vi "ColorProcessing2016_Custom2.vi"(11 "Original":T5=refnum) -> (0 "Blob array":T2(array[cluster])=[{"Area"=410.0, "Object Info"={"Object Center"={"X"=155.50975, "Y"=158.86829}, "Bounding Box"={"X Left"=142, "Y Top"=150, "X Right"=169, "Y Bottom"=168}, "Area"=410.0, "Orientation"=9.943739, "Aspect Ratio"=1.5, "Nb Holes"=0}}], 1 "Masked":T5(plugin-control), 2 "Targets":T4[](array[typedef]), 3 "Original Image":T5(plugin-control), 4 "Scored Particle Info 2":T1(array[cluster]))   [LabVIEW 2015]
uses:
  Camera Types.ctl
  <vilib>/vision/Image Controls.llb/IMAQ Image.ctl
  Scores.ctl
  <vilib>/vision/NI_Vision_Development_Module.lvlib
panel:
  in  "Range":cluster{"Lower value":sgl, "Upper value":sgl}={"Lower value"=128.0, "Upper value"=255.0} {"Upper value" format="%.2f"; "Lower value" format="%.2f"}
  in  "Particle Count Limit":i32=3
  out "Scored Particle Info":T1(array[cluster])
  in  "Area Size Limit %":dbl=0.5
  in  "Settings":T3={"Objects"=0, "Threshold"=1, "Reject Border"=TRUE, "Fill Holes"=FALSE, "Min Object Size"=TRUE, "Min Size"=350, "Max Object Size"=TRUE, "Max Size"=700, "Show Search Area"=TRUE, "Show Center"=TRUE, "Show Bounding Box"=TRUE} {"Objects" items=["Bright Objects", "Dark Objects"]; "Threshold" min=1 max=999999999 step=1; "Max Size" min=1 max=999999999 step=1; "Min Size" min=1 max=999999999 step=1}
  out "Qualified Particles":i32=3
  out "Sorted Particle Scores":T6(array[cluster]) {"Center" format="%#_3g"; "Moment Factor" format="%#_3g"; "Aspect Ratio" format="%#_3g"; "Area to CH" format="%#_3g"; "X" format="%#_3g"; "Y" format="%#_3g"}
  out "Detected Targets":T7(array[cluster]) {"Normalized Rect"."Numeric 5" format="%#_2g"; "Normalized Rect"."Numeric 3" format="%#_2g"; "Normalized Rect"."Numeric 2" format="%#_2g"; "Normalized Rect"."Numeric" format="%#_2g"}
  in  "Aspect Ratio Fudge Factor":dbl=1.0
  out "Highest Avg Score":dbl=85.32840563115018 format="%#_3g"
  in  "Min Score Threshold":i32=70
  in  "Camera Type":T8=enum."MS HD3000 square"
  in  "ROI DescriptorEmphasize Limit Tests":bool=TRUE
  # "Density Profile"
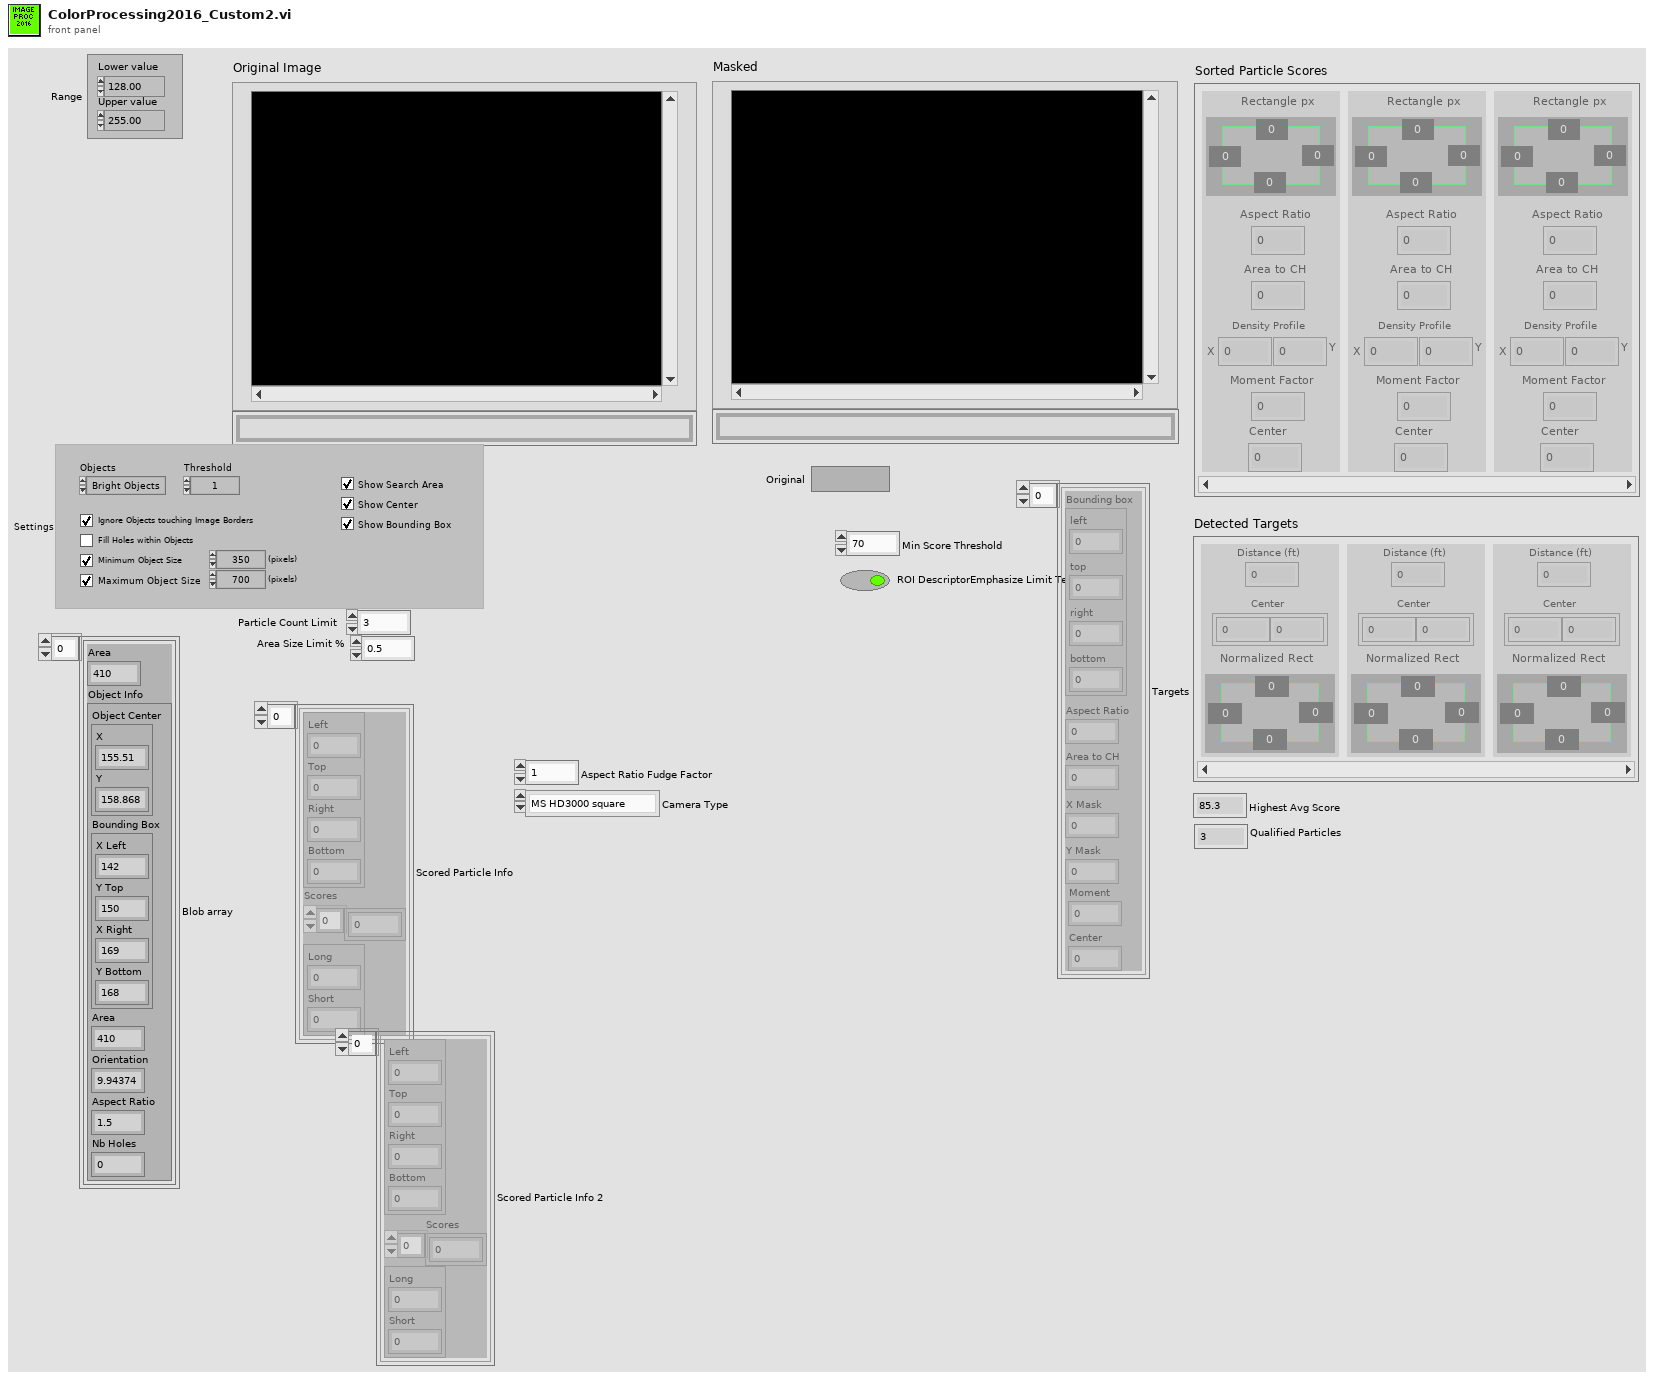
[diagram p1: front panel]
types:
  T1 = cluster{cluster{"Left":dbl, "Top":dbl, "Right":dbl, "Bottom":dbl}, "Scores":dbl[], cluster{"Long":dbl, "Short":dbl}}[]
  T2 = cluster{"Area":sgl, "Object Info":cluster{"Object Center":cluster{"X":sgl, "Y":sgl}, "Bounding Box":cluster{"X Left":i32, "Y Top":i32, "X Right":i32, "Y Bottom":i32}, "Area":sgl, "Orientation":sgl, "Aspect Ratio":sgl, "Nb Holes":i32}}[]
  T3 = cluster{"Objects":u16, "Threshold":i32, "Reject Border":bool, "Fill Holes":bool, "Min Object Size":bool, "Min Size":i32, "Max Object Size":bool, "Max Size":i32, "Show Search Area":bool, "Show Center":bool, "Show Bounding Box":bool}
  T4 = typedef "Scores.ctl" = cluster{"Bounding box":cluster{"left":dbl, "top":dbl, "right":dbl, "bottom":dbl}, "Aspect Ratio":dbl, "Area to CH":dbl, "X Mask":dbl, "Y Mask":dbl, "Moment":dbl, "Center":dbl}
  T5 = typedef "IMAQ Image.ctl" = refnum<image>
  T6 = cluster{"Rectangle px":cluster{"Numeric":dbl, "Numeric 2":dbl, "Numeric 3":dbl, "Numeric 5":dbl}, "Aspect Ratio":dbl, "Area to CH":dbl, "X":dbl, "Y":dbl, "Moment Factor":dbl, "Center":dbl}[]
  T7 = cluster{"Distance (ft)":dbl, "Center":cluster{dbl, dbl}, "Normalized Rect":cluster{"Numeric":dbl, "Numeric 2":dbl, "Numeric 3":dbl, "Numeric 5":dbl}}[]
  T8 = typedef "Camera Types.ctl" = enum16{"206", "1011", "1013", "MS HD3000 square", "MS HD3000 640x480"}
  T9 = typedef "Particle Parameters" = i32
  T10 = typedef "IMAQ Rectangle" = cluster{"Left":i32, "Top":i32, "Right":i32, "Bottom":i32, "Rotation":dbl}
  T11 = typedef "Image Type" = u32
  T12 = cluster{"Object Center":cluster{"X":sgl, "Y":sgl}, "Bounding Box":cluster{"X Left":i32, "Y Top":i32, "X Right":i32, "Y Bottom":i32}, "Area":sgl, "Orientation":sgl, "Aspect Ratio":sgl, "Nb Holes":i32}[]
  T13 = cluster{"Area":sgl, "Object Info":cluster{"Object Center":cluster{"X":sgl, "Y":sgl}, "Bounding Box":cluster{"X Left":i32, "Y Top":i32, "X Right":i32, "Y Bottom":i32}, "Area":sgl, "Orientation":sgl, "Aspect Ratio":sgl, "Nb Holes":i32}}
  T14 = cluster{"Rectangle":cluster{"Numeric":dbl, "Numeric 2":dbl, "Numeric 3":dbl, "Numeric 5":dbl}, "L":dbl, "Area to CH":dbl, "X":dbl, "Y":dbl, "Moment Factor":dbl, "Center":dbl}[]
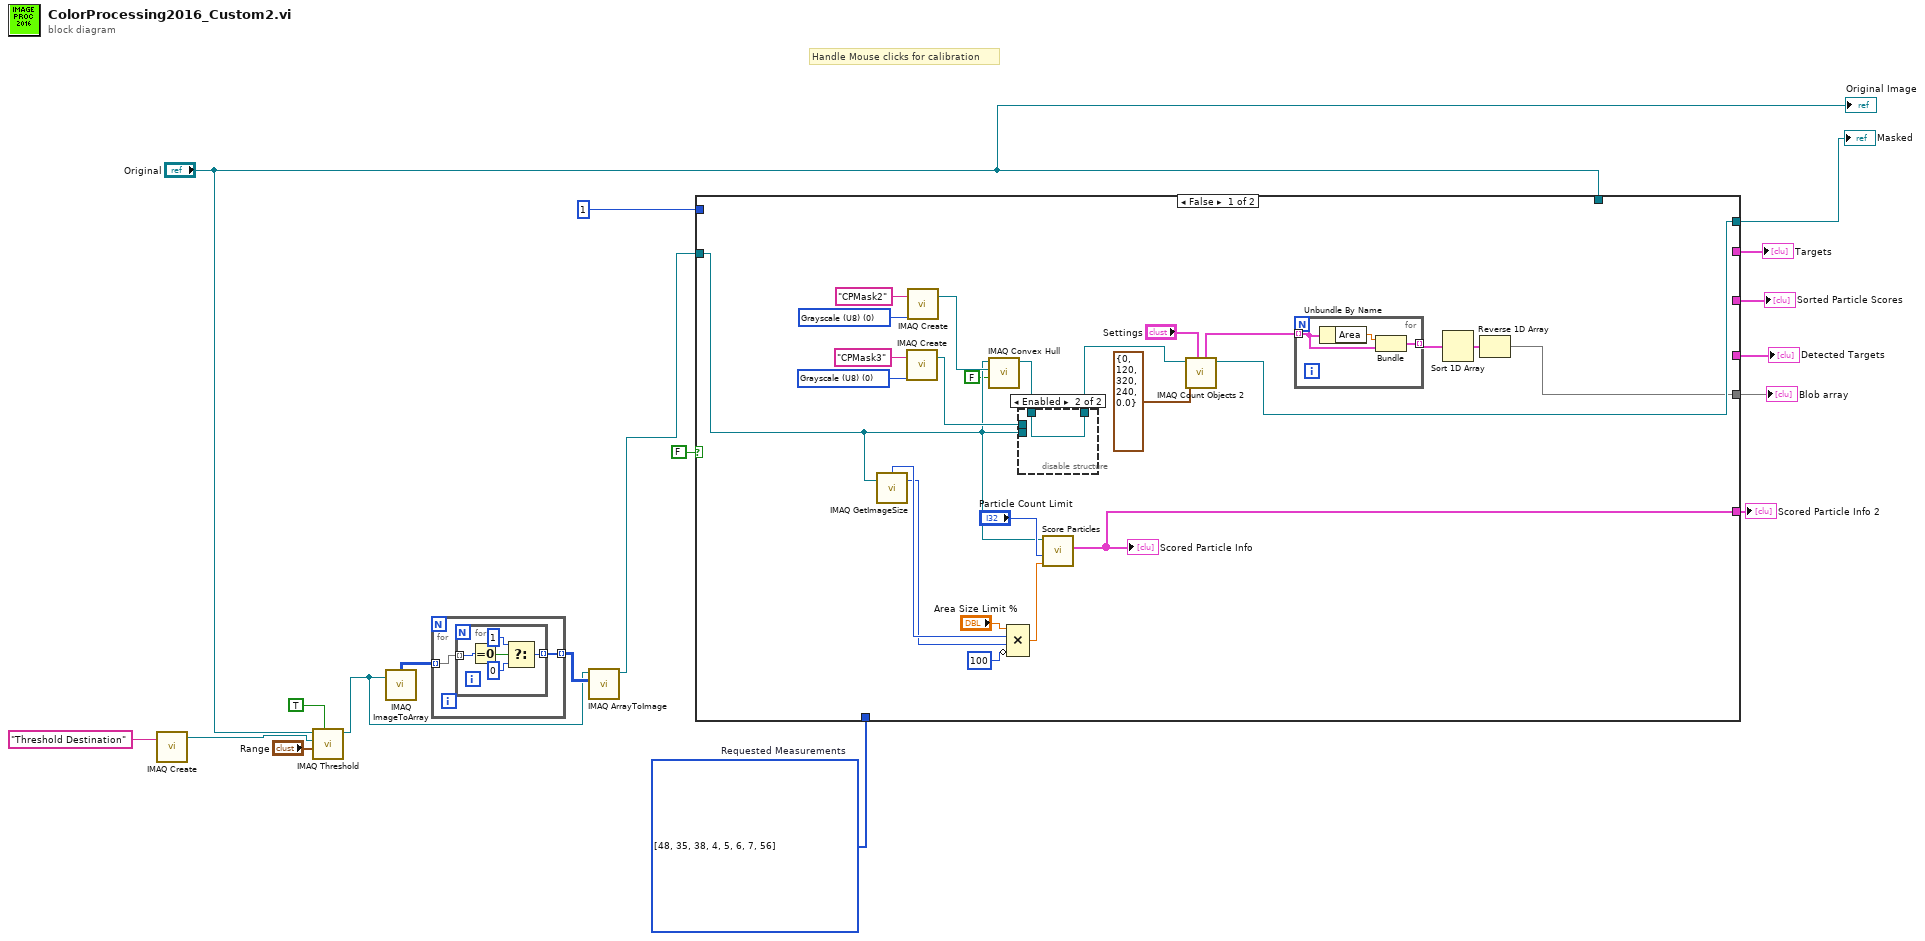
[diagram p0: block diagram]
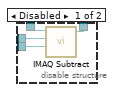
[diagram p2: hidden frame]
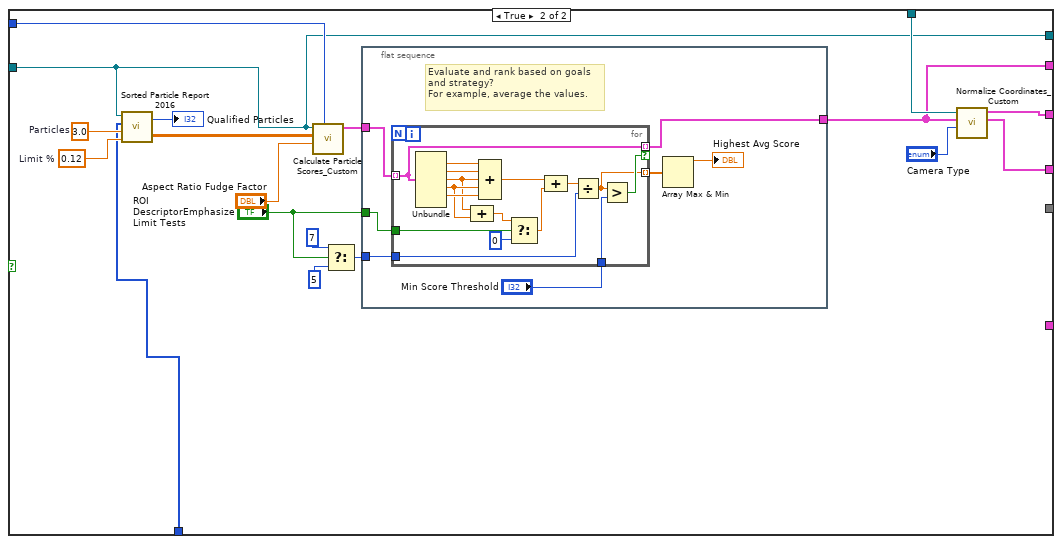
[diagram p3: hidden frame]
diagram:
  w11 = T9[] [48, 35, 38, 4, 5, 6, 7, 56] items=["Center of Mass X", "Center of Mass Y", "First Pixel X", "First Pixel Y", "Bounding Rect Left", "Bounding Rect Top", "Bounding Rect Right", "Bounding Rect Bottom", "Max Feret Diameter Start X", "Max Feret Diameter Start Y", "Max Feret Diameter End X", "Max Feret Diameter End Y", "Max Horiz. Segment Length Left", "Max Horiz. Segment Length Right", "Max Horiz. Segment Length Row", "-", "Bounding Rect Width", "Bounding Rect Height", "Bounding Rect Diagonal", "Perimeter", "Convex Hull Perimeter", "Holes' Perimeter", "Max Feret Diameter", "Equivalent Ellipse Major Axis", "Equivalent Ellipse Minor Axis", "Equivalent Ellipse Minor Axis (Feret)", "Equivalent Rect Long Side", "Equivalent Rect Short Side", "Equivalent Rect Diagonal", "Equivalent Rect Short Side (Feret)", "Average Horiz. Segment Length", "Average Vert. Segment Length", "Hydraulic Radius", "Waddel Disk Diameter", "-", "Area", "Holes' Area", "Particle & Holes' Area", "Convex Hull Area", "Image Area", "-", "Number of Holes", "Number of Horiz. Segments", "Number of Vert. Segments", "-", "Orientation", "Max Feret Diameter Orientation", "-", "% Area/Image Area", "% Area/(Particle & Holes' Area)", "Ratio of Equivalent Ellipse Axes", "Ratio of Equivalent Rect Sides", "-", "Elongation Factor", "Compactness Factor", "Heywood Circularity Factor", "Type Factor", "-", "Sum X", "Sum Y", "Sum XX", "Sum XY", "Sum YY", "Sum XXX", "Sum XXY", "Sum XYY", "Sum YYY", "-", "Moment of Inertia XX", "Moment of Inertia XY", "Moment of Inertia YY", "Moment of Inertia XXX", "Moment of Inertia XXY", "Moment of Inertia XYY", "Moment of Inertia YYY", "Norm. Moment of Inertia XX", "Norm. Moment of Inertia XY", "Norm. Moment of Inertia YY", "Norm. Moment of Inertia XXX", "Norm. Moment of Inertia XXY", "Norm. Moment of Inertia XYY", "Norm. Moment of Inertia YYY", "Hu Moment 1", "Hu Moment 2", "Hu Moment 3", "Hu Moment 4", "Hu Moment 5", "Hu Moment 6", "Hu Moment 7"]  # Requested Measurements
  # "Handle Mouse clicks for calibration"
  n1 = call "IMAQ Create"("Image Name"="Threshold Destination") -> ("New Image"=w3:T5)  [unwired: 4 in, 1 out]
  n2 = call "IMAQ Threshold"("Keep/Replace Value (Replace)"=TRUE, "Range"="Range", "Image Dst"=w3, "Image Src"="Original") -> ("Image Dst Out"=w5:T5)  [unwired: 6 in, 1 out]
  n3 = call "IMAQ ImageToArray"("Image"=w5) -> ("Image Pixels (U8)"=w7:u8[][])  [unwired: 3 in, 4 out]
  n4 = for {
    tunnel: w7 -> [w20] mode=indexing
    tunnel: [w19] -> w6 mode=indexing
    n5 = for {
      tunnel: w20 -> [w25] mode=indexing
      tunnel: [w21] -> w19 mode=indexing
      n6 = Equal To 0?(x=w25) -> (x = 0?=w24:bool)
      n7 = Select(t=u8 1, s=w24, f=u8 0) -> (s? t:f=w21:u8)
    }
  }
  n8 = call "IMAQ ArrayToImage"("Image Pixels (U8)"=w6, "Image"=w5) -> ("Image Out"=w2:T5)  [unwired: 8 in, 1 out]
  n9 = case shown="False" FALSE {
    tunnel: [_ w68] -> w18
    tunnel: 1 ("Replace Value") -> [_ w67]
    tunnel: "Original" -> [_ w62]
    tunnel: [_ w61] -> w16
    tunnel: [_ w60] -> w15
    tunnel: w2 -> [w29 w59]
    tunnel: [w38 w59] -> w14
    tunnel: [w37 _] -> w13
    tunnel: w11 -> [_ w58]
    tunnel: [w30 _] -> w10
    frame False {
      w44 = T11 0 items=["Grayscale (U8)", "Grayscale (I16)", "Grayscale (SGL)", "Complex (CSG)", "RGB (U32)", "HSL (U32)", "RGB (U64)", "Grayscale (U16)"] ("Image Type")
      w42 = T11 0 items=["Grayscale (U8)", "Grayscale (I16)", "Grayscale (SGL)", "Complex (CSG)", "RGB (U32)", "HSL (U32)", "RGB (U64)", "Grayscale (U16)"] ("Image Type")
      n10 = call "IMAQ GetImageSize"("Image"=w29) -> ("Y Resolution"=w27:i32, "X Resolution"=w28:i32)  [unwired: 3 in, 1 out]
      n11 = call "IMAQ Create"("Image Name"="CPMask3", "Image Type"=w44) -> ("New Image"=w46:T5)  [unwired: 2 in, 2 out]
      n12 = call "IMAQ Create"("Image Name"="CPMask2", "Image Type"=w42) -> ("New Image"=w43:T5)  [unwired: 2 in, 2 out]
      n13 = call "IMAQ Convex Hull"("Connectivity 4/8 (8)"=FALSE, "Image Dst"=w43, "Image Src"=w29) -> ("Image Dst Out"=w36:T5)  [unwired: 7 in, 1 out]
      n14 = Compound Arithmetic op=MULTIPLY("Area Size Limit %", w28, w27, invert 100 ("length")) -> (w31:dbl)
      n15 = disable-structure shown="Enabled" {
        disable-tunnel: w46 -> [w53 _]
        disable-tunnel: w29 -> [w52 _]
        disable-tunnel: w36 -> [w51 w54]
        disable-tunnel: [w50 w54] -> w35
        frame Disabled {
          n16 = call "IMAQ Subtract"("Image Src A"=w51, "Image Dst"=w53, "Image Src B"=w52) -> ("Image Dst Out"=w50:T5)  [unwired: 4 in, 1 out]
        }
        frame Enabled {
        }
      }
      n17 = call "Score Particles.vi"("Area Size Limit"=w31, "Particle Count Limit"="Particle Count Limit", "Image Refnum in"=w29) -> ("Scored Particle Info"=w30:T1)  [unwired: 7 in, 1 out]
      "Scored Particle Info" <- w30
      n18 = call "IMAQ Count Objects 2"("Settings"="Settings", "Search Rect (entire image)"=T10 {"Left"=0, "Top"=120, "Right"=320, "Bottom"=240, "Rotation"=0.0}, "Image"=w35) -> ("Image Out"=w38:T5, "Objects"=w47:T12)  [unwired: 4 in, 3 out]
      n19 = for {
        tunnel: w47 -> [w57] mode=indexing
        tunnel: [w55] -> w48 mode=indexing
        n20 = Unbundle By Name(w57) -> ("Area"=w56:sgl)
        n21 = Bundle("Area"=w56, "Object Info"=w57) -> (w55:T13)  [unwired: 1 in]
      }
      n22 = Sort 1D Array(array=w48) -> (sorted array=w49:T2)
      n23 = Reverse 1D Array(array=w49) -> (reversed array=w37:T2)
    }
    frame True {
      w66 = 0.12  # Limit %
      w63 = 3.0  # Particles
      n24 = call "Sorted Particle Report 2016.vi"("Min Area Size %"=w66, "Particle Count Limit"=w63, "Pixel Measurements"=w58, "Image in"=w59) -> ("Sorted Data"=w65:dbl[][], "Particles"=→"Qualified Particles":i32)
      n25 = call "Calculate Particle Scores_Custom.vi"("Pixel Value"=w67, "Aspect Fudge Factor"="Aspect Ratio Fudge Factor", "Sorted Data"=w65, "Image in"=w59) -> ("Scores"=w70:T4[])  [unwired: 7 in]
      n26 = Select(t=7, s="ROI DescriptorEmphasize Limit Tests", f=5) -> (s? t:f=w74:i32)
      n27 = flat-sequence {
        tunnel: w70 -> [w81]
        tunnel: [w82] -> w61
        tunnel: w74 -> [w78]
        tunnel: "ROI DescriptorEmphasize Limit Tests" -> [w76]
        frame #0 {
          # "Evaluate and rank based on goals\nand strategy?\nFor example, average the values."
          n28 = for {
            tunnel: w81 -> [w96] mode=indexing
            tunnel: [w96] -> w82 mode=indexing if=w95
            tunnel: [w94] -> w80 mode=indexing
            tunnel: w78 -> [w93]
            tunnel: "Min Score Threshold" -> [w92]
            tunnel: w76 -> [w85]
            n29 = Unbundle(w96) -> ("Aspect Ratio"=w98:dbl, "Area to CH"=w97:dbl, "X Mask"=w87:dbl, "Y Mask"=w88:dbl, "Moment"=w89:dbl)  [unwired: 2 out]
            n30 = Compound Arithmetic op=ADD(w87, w88) -> (w86:dbl)
            n31 = Compound Arithmetic op=ADD(w98, w97, w87, w88, w89) -> (w91:dbl)
            n32 = Select(t=w86, s=w85, f=0) -> (s? t:f=w84:dbl)
            n33 = Compound Arithmetic op=ADD(w91, w84) -> (w90:dbl)
            n34 = Divide(x=w90, y=w93) -> (x/y=w94:dbl)
            n35 = Greater?(x=w94, y=w92) -> (0:w95:bool)
          }
          n36 = Array Max & Min(array=w80) -> (max value=→"Highest Avg Score":dbl)  [unwired: 3 out]
        }
      }
      n37 = call "Normalize Coordinates_Custom.vi"("Camera Type"="Camera Type", "Targets"=w61, "Image in"=w62) -> ("Found Targets"=w68:T7, "Sorted Scores"=w60:T14)  [unwired: 7 in]
    }
  }
  "Masked" <- w14
  "Sorted Particle Scores" <- w15
  "Detected Targets" <- w18
  "Targets" <- w16
  "Blob array" <- w13
  "Scored Particle Info 2" <- w10
  "Original Image" <- "Original"
